vi "initializeArrayElement.vi"(8 "error in (no error)":errorcluster, 9 "arraySize":u16, 10 "arrayRef":refnum<vi>, 11 "Enum in":refnum<class "Enum.lvclass">) -> (0 "error out":errorcluster, 3 "Enum out":refnum<class "Enum.lvclass">)   [LabVIEW 2016, in "Enum.lvclass"]
uses:
  Enum.lvclass
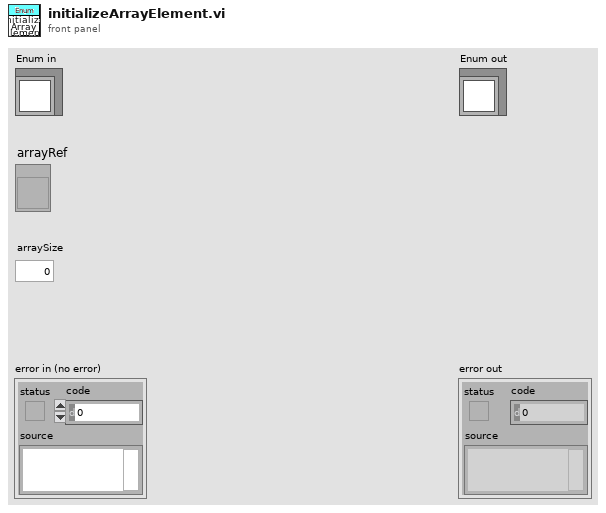
[diagram p1: front panel]
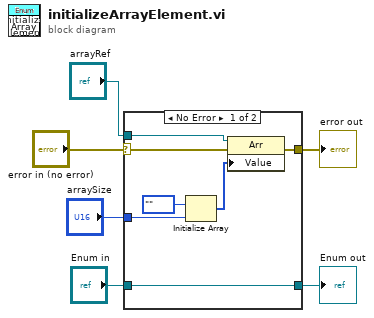
[diagram p0: block diagram]
diagram:
  n1 = case shown="No Error" "error in (no error)" {
    selector: "error in (no error)" -> [w12 w15]
    tunnel: [w11 w15] -> w3
    tunnel: "arraySize" -> [w10 _]
    tunnel: "arrayRef" -> [w9 _]
    tunnel: "Enum in" -> [w8 w14]
    tunnel: [w8 w14] -> w5
    frame No Error {
      n2 = Initialize Array(enum32{""}."", w10) -> (w13:enum32{""}[])
      n3 = property class="Arr"(reference=w9, error in=w12, "Value"=w13) -> (error out=w11:errorcluster)  [unwired: 1 out]
    }
    frame Error {
    }
  }
  "error out" <- w3
  "Enum out" <- w5
